vi "DAC Configure.vi"(8 "error in":errorcluster, 11 "DAC Jumo DP in":refnum<class "DAC Jumo DP.lvclass">) -> (0 "error out":errorcluster, 3 "DAC Jumo DP out":refnum<class "DAC Jumo DP.lvclass">)   [LabVIEW 2019, in "DAC.lvlib" / "DAC Jumo DP.lvclass"]
uses:
  DAC Jumo DP.lvclass
  C:/Users/wg/Documents/LV_Projects/test-stand/App/DAC/DAC.lvclass
  DAC.lvclass/DAC.ctl
  DAC Jumo DP.lvclass/DAC Jumo DP.ctl
  DAC.lvclass
  <resource>/objmgr/daqmx.rc
  <vilib>/DAQmx/create/channels.llb/DAQmx Create Channel (AI-Voltage-Basic).vi
  <vilib>/DAQmx/create/scale.llb/DAQmx Create Scale (Map Ranges).vi
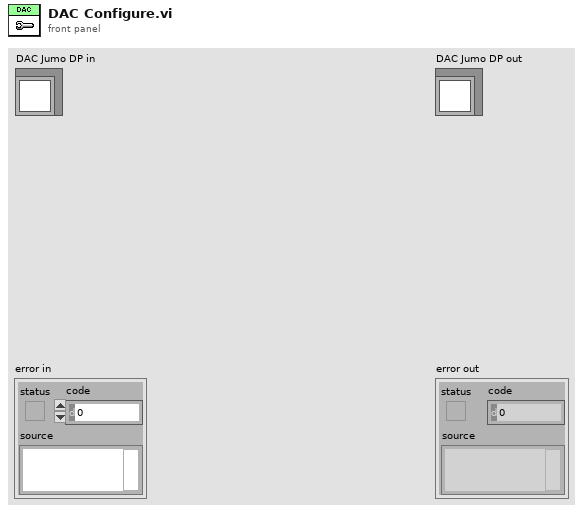
[diagram p1: front panel]
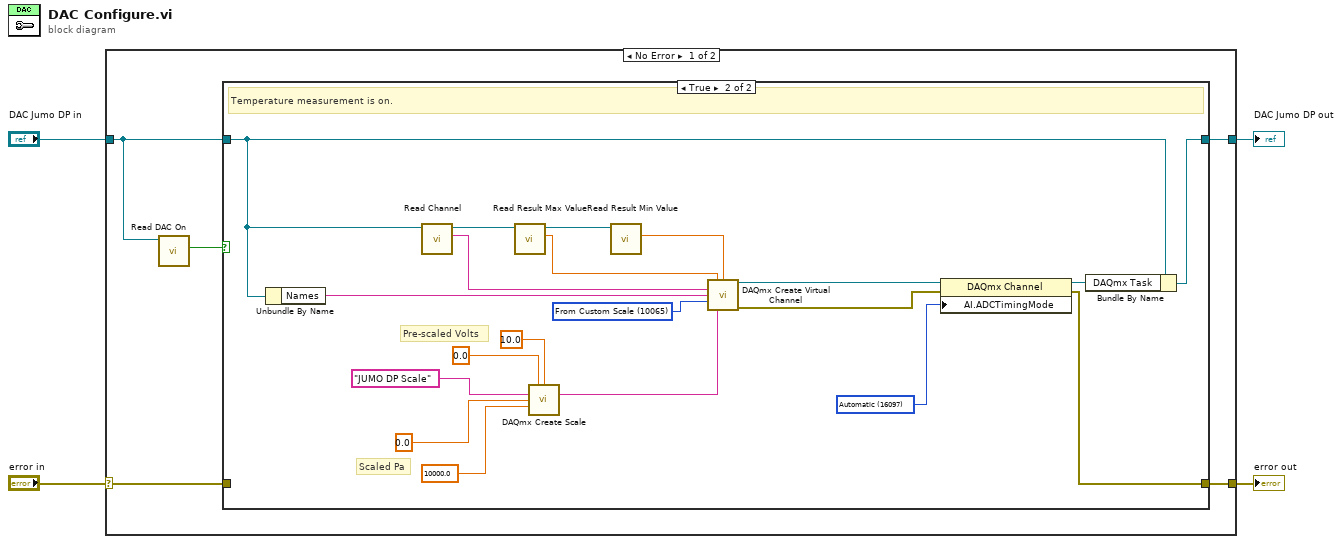
[diagram p0: block diagram]
diagram:
  n1 = case shown="No Error" "error in" {
    selector: "error in" -> [w6 w33]
    tunnel: [w5 w33] -> w4
    tunnel: [w7 w32] -> w3
    tunnel: "DAC Jumo DP in" -> [w9 w32]
    frame No Error {
      n2 = call "Read DAC On.vi"("DAC in"=w9) -> ("DAC On"=w8:bool)  [unwired: 8 in, 2 out]
      n3 = case shown="True" w8 {
        tunnel: w9 -> [w11 w26]
        tunnel: [w11 w31] -> w7
        tunnel: w6 -> [w10 _]
        tunnel: [w10 w19] -> w5
        frame False {
          # "Temperature measurement is off."
        }
        frame True {
          w18 = 10065 items=["Volts"=10348, "From Custom Scale"=10065] ("units")
          w27 = 16097 items=["Automatic"=16097, "High Resolution"=10195, "High Speed"=14712, "Best 50 Hz Rejection"=14713, "Best 60 Hz Rejection"=14714, "Custom"=10137] ("AI.ADCTimingMode")
          # "Scaled Pa"
          # "Pre-scaled Volts"
          # "Temperature measurement is on."
          n4 = Unbundle By Name(w26) -> ("Names"=w30:string)
          n5 = call "Read Channel.vi"("DAC in"=w26) -> ("Channel"=w25:string, "DAC out"=w24:refnum<class "DAC Jumo DP.lvclass">)  [unwired: 8 in, 1 out]
          n6 = call "Read Result Max Value.vi"("DAC in"=w24) -> ("Max Value"=w21:dbl, "DAC out"=w23:refnum<class "DAC Jumo DP.lvclass">)  [unwired: 8 in, 1 out]
          n7 = call-poly <vilib>:"DAQmx Create Scale.vi"("pre-scaled minimum"=0.0, "pre-scaled maximum"=10.0, "name"="JUMO DP Scale", "scaled minimum"=0.0, "scaled maximum"=10000.0) -> ("scale out"=w12:tag)  [unwired: 9 in, 1 out]
          n8 = call "Read Result Min Value.vi"("DAC in"=w23) -> ("Min Value"=w22:dbl)  [unwired: 8 in, 2 out]
          n9 = call-poly <vilib>:"DAQmx Create Virtual Channel.vi"("maximum value"=w21, "minimum value"=w22, "physical channels"=w25, "name to assign"=w30, "units"=w18, "custom scale name"=w12) -> ("task out"=w29:refnum<k21>, "error out"=w20:errorcluster)  [unwired: 8 in]
          n10 = property class="DAQmx Channel"(reference=w29, error in=w20, "AI.ADCTimingMode"=w27) -> (reference out=w28:refnum<k21>, error out=w19:errorcluster)
          n11 = Bundle By Name(cluster=w26, "DAQmx Task"=w28) -> (w31:refnum<class "DAC Jumo DP.lvclass">)
        }
      }
    }
    frame Error {
    }
  }
  "error out" <- w4
  "DAC Jumo DP out" <- w3
